vi "DFConfig Open My.Datafinder.vi"(8 "error in (no error)":errorcluster, 11 "my.datafinder Path (empty)":path) -> (0 "error out":errorcluster, 3 "my.datafinder":string)   [LabVIEW 2011]
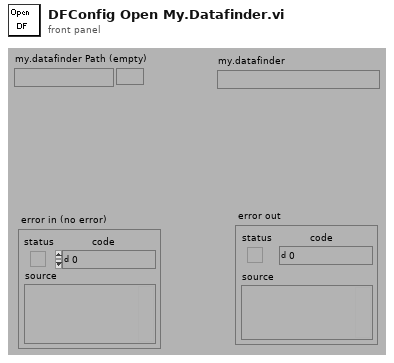
[diagram p1: front panel]
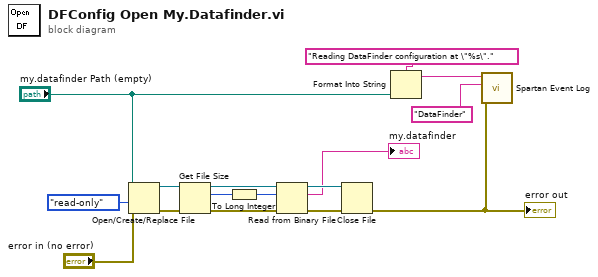
[diagram p0: block diagram]
diagram:
  n1 = Open/Create/Replace File(file path (use dialog)="my.datafinder Path (empty)", error in="error in (no error)", access (0:read/write)=enum16{"read/write", "read-only", "write-only"}."read-only") -> (refnum out=w14:refnum<file>, error out=w12:errorcluster)  [unwired: 4 out]
  n2 = Get File Size(file=w14, error in=w12) -> (refnum out=w13:refnum<file>, size (in bytes)=w10:i64, 0:w11:errorcluster)
  n3 = To Long Integer(number=w10) -> (32bit integer=w9:i32)
  n4 = Read from Binary File(8:w11, 10:w9, 11:w13) -> (0:w15:errorcluster, 2:→"my.datafinder":string, 3:w16:refnum<file>)  [unwired: 4 out]
  n5 = Close File(refnum=w16, error in=w15) -> (error out=w2:errorcluster)  [unwired: 1 out]
  "error out" <- w2
  n6 = Format Into String(format string="Reading DataFinder configuration at \"%s\".", "my.datafinder Path (empty)") -> (resulting string=w4:string)  [unwired: 2 in, 1 out]
  n7 = call "Spartan Event Log.vi"("error in (no error)"=w2, "module (\"\")"="DataFinder" ("module (\"\")"), "message (\"\")"=w4) -> ()  [unwired: 2 in, 4 out]
